vi "ReadAppKey.vi"(10 "Reset":bool) -> (2 "APIKey":string)   [LabVIEW 2019]
panel:
  # "To make this work, you have to have moved your\nibm-credentials.env file into your LabVIEW Data:AppKey Files\nfolder"
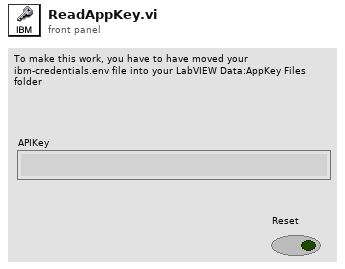
[diagram p1: front panel]
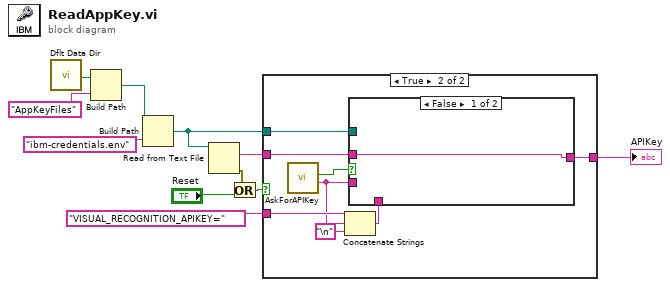
[diagram p0: block diagram]
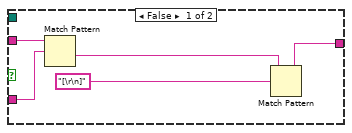
[diagram p2: hidden frame]
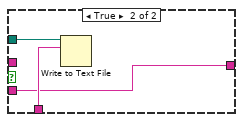
[diagram p3: hidden frame]
diagram:
  n1 = call <vilib>:"Dflt Data Dir.vi"() -> ("App:Default Data Directory"=w9:path)
  n2 = Build Path(base path=w9, name or relative path="AppKeyFiles") -> (appended path=w8:path)
  n3 = Build Path(base path=w8, name or relative path="ibm-credentials.env") -> (appended path=w5:path)
  n4 = Read from Text File(file (use dialog)=w5) -> (text=w4:string, error out=w3:errorcluster)  [unwired: 3 in, 2 out]
  n5 = Or(x=w3, y="Reset") -> (x .or. y?=w1:bool)
  n6 = case shown="True" w1 {
    tunnel: w4 -> [w16 w17]
    tunnel: "VISUAL_RECOGNITION_APIKEY=" -> [w15 w22]
    tunnel: [w12 w24] -> w6
    tunnel: w5 -> [_ w23]
    frame False {
      n7 = Match Pattern(string=w16, regular expression=w15) -> (after substring=w14:string)  [unwired: 1 in, 3 out]
      n8 = Match Pattern(string=w14, regular expression="[\r\n]") -> (before substring=w12:string)  [unwired: 1 in, 3 out]
    }
    frame True {
      n9 = call "AskForAPIKey.vi"() -> ("String out"=w18:string, "success?"=w19:bool)  [unwired: 9 in, 1 out]
      n10 = Concatenate Strings(w22, w18, "\n" ("string")) -> (w20:string)
      n11 = case shown="False" w19 {
        tunnel: [w25 w26] -> w24
        tunnel: w23 -> [_ w28]
        tunnel: w20 -> [_ w27]
        tunnel: w18 -> [_ w26]
        tunnel: w17 -> [w25 _]
        frame False {
        }
        frame True {
          n12 = Write to Text File(file (use dialog)=w28, text=w27) -> ()  [unwired: 2 in, 3 out]
        }
      }
    }
  }
  "APIKey" <- w6
